vi "Connect Core.vi"(4 "queueRef":refnum<queue>, 5 "Commit Only?":bool, 6 "Access (R/W allowed)":T1, 7 "Mode (buffer)":u16(ring)=1 items=["commit", "buffer"], 8 "Error In":errorcluster, 11 "SVConnection in":refnum<class "SVConnection.lvclass">) -> (0 "Error Out":errorcluster, 3 "SVConnection out":refnum<class "SVConnection.lvclass">)   [LabVIEW 2015, in "CS++SharedVariables.lvlib" / "SVConnection.lvclass"]
doc: "Open reference to a shared variable if not already connected."
uses:
  SVConnection.lvclass
  SVConnection.lvclass/SVConnection.ctl
  CS++BaseClasses/Base/CS++Base.lvclass/CS++Base.ctl
  PVConnection/PVConnection.lvclass/PVConnection.ctl
  ProcessVariable/PV.lvclass/PV.ctl
  ProcessVariable/PV.lvclass
  PVConnection/PVConnection.lvclass
  Libraries/Utilities/CS++Utilities.lvlib
  CS++BaseClasses/Base/CS++Base.lvclass
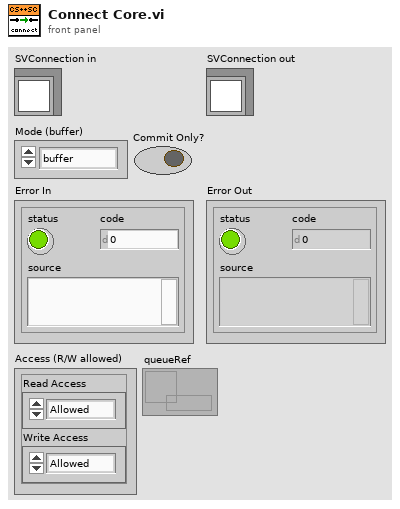
[diagram p1: front panel]
types:
  T1 = cluster{"Read Access":enum8{"Allowed", "Required", "None"}, "Write Access":enum8{"Allowed", "Required", "None"}}
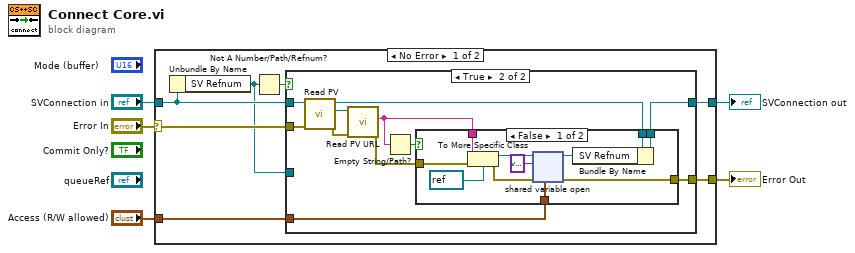
[diagram p0: block diagram]
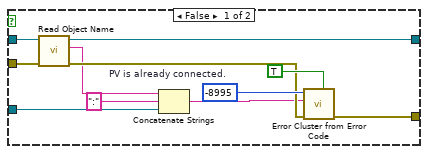
[diagram p2: hidden frame]
diagram:
  n1 = case shown="No Error" "Error In" {
    selector: "Error In" -> [w12 w49]
    tunnel: [w11 w49] -> w4
    tunnel: [w10 w48] -> w2
    tunnel: "SVConnection in" -> [w7 w48]
    tunnel: "Access (R/W allowed)" -> [w8 _]
    frame No Error {
      n2 = Unbundle By Name(w7) -> ("SV Refnum"=w6:refnum<k21>)
      n3 = Not A Number/Path/Refnum?(number/path/refnum=w6) -> (NaN/Path/Refnum?=w9:bool)
      n4 = case shown="True" w9 {
        tunnel: w12 -> [w18 w27]
        tunnel: [w23 w34] -> w11
        tunnel: [w19 w33] -> w10
        tunnel: w7 -> [w20 w31]
        tunnel: w8 -> [_ w32]
        tunnel: w6 -> [w14 _]
        frame False {
          w21 = -8995  # PV is already connected.
          n5 = call "Read Object Name.vi"("error in (no error)"=w18, "Base in"=w20) -> ("error out"=w17:errorcluster, "Object Name"=w16:string, "Base out"=w19:refnum<class "SVConnection.lvclass">)  [unwired: 7 in]
          n6 = Concatenate Strings(w16, ":" ("string"), w14) -> (w13:string)
          n7 = call "Error Cluster from Error Code.vi"("is warning? (False)"=TRUE ("show call chain? (False)"), "Error In"=w17, "Error Message (\"\")"=w13, "Error Code (0)"=w21) -> ("Error Out"=w23:errorcluster)  [unwired: 7 in]
        }
        frame True {
          n8 = call "Read PV.vi"("error in (no error)"=w27, "PVConnection in"=w31) -> ("error out"=w29:errorcluster, "PV"=w30:refnum<class "PV.lvclass">, "PVConnection out"=w26:refnum<class "SVConnection.lvclass">)  [unwired: 7 in]
          n9 = call "Read PV URL.vi"("error in (no error)"=w29, "PV in"=w30) -> ("error out"=w28:errorcluster, "PV URL"=w25:string)  [unwired: 7 in, 1 out]
          n10 = Empty String/Path?(string/path=w25) -> (empty?=w24:bool)
          n11 = case shown="False" w24 {
            tunnel: [w41 w47] -> w34
            tunnel: [w39 w46] -> w33
            tunnel: w32 -> [w38 _]
            tunnel: w25 -> [w37 _]
            tunnel: w28 -> [w36 w47]
            tunnel: w26 -> [w35 w46]
            frame False {
              n12 = To More Specific Class(target class=refnum<k21> refnum ("shared variable refnum in"), reference=w37, error in=w36) -> (specific class reference=w44:refnum<k21>, error out=w43:errorcluster)
              n13 = shared-variable-open(w44, w43, variant ("variant"), w38) -> (w40:refnum<k21>, w41:errorcluster)
              n14 = Bundle By Name(cluster=w35, "SV Refnum"=w40) -> (w39:refnum<class "SVConnection.lvclass">)
            }
            frame True {
            }
          }
        }
      }
    }
    frame Error {
    }
  }
  "Error Out" <- w4
  "SVConnection out" <- w2
